vi "JKISM++ Convert HexStr to Data.vi"(2 "HEX String":string) -> (7 "Variant":variant, 9 "error out":errorcluster)   [LabVIEW 2014, in "JKI State Machine++.lvlib"]
doc: "Convert hex string arguments back to variant.\n\n<b>Inputs:</b>\n - <b>HEX String</b>: Hex String, which contains no invisible string following JKISM's rule\n\n<b>Outputs:</b>\n - <b>Variant</b>: Complex data in variant format.\n - <b>error out</b>: Error output"
uses:
  JKI State Machine++.lvlib
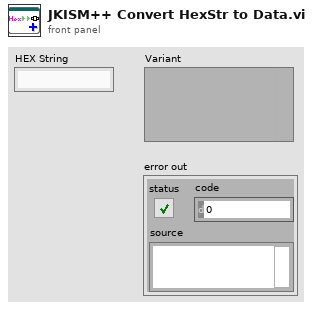
[diagram p1: front panel]
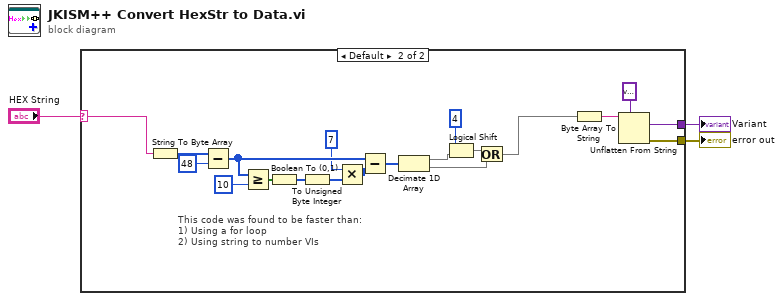
[diagram p0: block diagram]
diagram:
  n1 = case shown="Default" "HEX String" {
    selector: "HEX String" -> [_ w6]
    tunnel: [_ w22] -> w3
    tunnel: [_ w4] -> w1
    frame "" {
    }
    frame Default {
      # "This code was found to be faster than:\n1) Using a for loop\n2) Using string to number VIs"
      n2 = String To Byte Array(string=w6) -> (unsigned byte array=w7:u8[])
      n3 = Subtract(x=w7, y=u8 48) -> (x-y=w18:u8[])
      n4 = Greater Or Equal?(x=w18, y=u8 10) -> (x >= y?=w15:bool[])
      n5 = Boolean To (0,1)(Boolean=w15) -> (0, 1=w13:i16[])
      n6 = To Unsigned Byte Integer(number=w13) -> (unsigned 8bit integer=w16:u8[])
      n7 = Multiply(x=u8 7, y=w16) -> (x*y=w17:u8[])
      n8 = Subtract(x=w18, y=w17) -> (x-y=w9:u8[])
      n9 = Decimate 1D Array(w9) -> (w10:u8[], w8:u8[])
      n10 = Logical Shift(y=i8 4, x=w10) -> (x << y=w19:u8[])
      n11 = Or(x=w19, y=w8) -> (x .or. y?=w5:u8[])
      n12 = Byte Array To String(unsigned byte array=w5) -> (string=w21:string)
      n13 = Unflatten From String(type=variant, binary string=w21) -> (value=w22:variant, error out=w4:errorcluster)  [unwired: 3 in, 1 out]
    }
  }
  "Variant" <- w3
  "error out" <- w1
